vi "CG-Test.vi"() -> ()   [LabVIEW 2020, in "Erweiterte Konfig.lvlib" / "CG-Check Konfig.lvlib"]
uses:
  CG-Check Konfig.lvlib
  Visualisierungs Elemente/String - Ausgabefeld.ctl
  Aktion_CG-Check.ctl
  Aktion_CG-Check_Protokoll.ctl
  CalEingaenge.ctl
  Zustand CG-Check.ctl
  Funktionstasten/Funktionstasten-Aktion.ctl
  Funktionstasten/Zustaende.ctl
  CalGas Aufschaltung/FGV CalGas Aktionen.ctl
  Stoerungen/Stoerungen Messgeraet/Aktionen Kommunikation Stoerung.ctl
  FT-IR/FGV FT-IR Gasliste Aktionen.ctl
  Funktionstasten/Freigabe Aktionen.ctl
  Funktionstasten/Funktionstasten.lvlib
  Stoerungen/Stoerungen.lvlib
  Allgemein/allgemeine Sub-VIs.lvlib
  FT-IR/FT-IR.lvlib
  CalGas Aufschaltung/CalGas Aufschaltung.lvlib
panel:
  out "Anzeige 6":string
  out "Istwert 6":sgl format="%#.2f"
  out "Ist\nAbweichung":T1 {"Abweichung 6" format="%#_5g"; "Abweichung 5" format="%#_5g"; "Abweichung 4" format="%#_5g"; "Abweichung 3" format="%#_5g"; "Abweichung 2" format="%#_5g"; "Abweichung 1" format="%#_5g"}
  out "Span Gas":string
  out "Komponenten":T2 {"Komponente 6" items=["---", "NO (350,3000) LP 191C", "NO2 (150) LP 191C (1of2)", "NO2 (2000) LP 191C (2of2)", "N2O (300) LP 191C (1of2)", "NH3 (300) LP 191C (1of2)", "NH3 (900,3000) LP 191C (2of2)", "HNCO (400) 191C", "H2O% (30) LP 191C", "Formaldehyde (70,500) LP 191C", "CO2 low% (4) LP 191C (2of2)", "CO2% (20) LP 191C (1of2)", "CO (700) LP 191C (1of3)", "CO% (1) LP 191C (2of3)", "Propylene (1000) LP 191C", "Aromatic HC C7 (500) LP 191C", "Ethylene (1000) LP 191C", "CH4 (250) LP 191C (1of2)", "CH4 (5000) LP 191C (2of2)", "Ethane (1000) LP 191C", "Acetylene (1000) LP 191C", "HNO2 (20) 191C", "MeOH (1000) 191C", "CO% (10) LP 191C (3of3)", "Formic Acid (100) 191C", "SO2 (500) LP 191C", "Acetaldehyde (1000) LP 191C", "COS (100) LP 191C", "1,3 butadiene (100) LP 191C", "Oil as Octane (200) LP 191C", "N2O (1000) LP 191C (2of2)", "Propane (200) LP 191C", "NO2 autorange (2000)", "CO autorange (100000)", "CH4 autorange (5000)", "NH3 autorange (3000)", "NOx autorange (3000)", "HCD (10000)", "NMHCD (10000)", "CO2% autorange (20)", "H2Oppm (300000)", "N2O autorange (1000)", "NMNEHCD (3000)", "FEQTHC ppmC1", "Temp. Gascell", "Pressure Gascell", "sBeam@2500", "Temp. HL to FT-IR", "Temp. HL Extern SP1", "Outlet Temp FT-IR", "Temp. Cabinet", "Constant 0", "Constant 50", "Constant 100", "AK DUMMY"]; "Komponente 5" items=["---", "NO (350,3000) LP 191C", "NO2 (150) LP 191C (1of2)", "NO2 (2000) LP 191C (2of2)", "N2O (300) LP 191C (1of2)", "NH3 (300) LP 191C (1of2)", "NH3 (900,3000) LP 191C (2of2)", "HNCO (400) 191C", "H2O% (30) LP 191C", "Formaldehyde (70,500) LP 191C", "CO2 low% (4) LP 191C (2of2)", "CO2% (20) LP 191C (1of2)", "CO (700) LP 191C (1of3)", "CO% (1) LP 191C (2of3)", "Propylene (1000) LP 191C", "Aromatic HC C7 (500) LP 191C", "Ethylene (1000) LP 191C", "CH4 (250) LP 191C (1of2)", "CH4 (5000) LP 191C (2of2)", "Ethane (1000) LP 191C", "Acetylene (1000) LP 191C", "HNO2 (20) 191C", "MeOH (1000) 191C", "CO% (10) LP 191C (3of3)", "Formic Acid (100) 191C", "SO2 (500) LP 191C", "Acetaldehyde (1000) LP 191C", "COS (100) LP 191C", "1,3 butadiene (100) LP 191C", "Oil as Octane (200) LP 191C", "N2O (1000) LP 191C (2of2)", "Propane (200) LP 191C", "NO2 autorange (2000)", "CO autorange (100000)", "CH4 autorange (5000)", "NH3 autorange (3000)", "NOx autorange (3000)", "HCD (10000)", "NMHCD (10000)", "CO2% autorange (20)", "H2Oppm (300000)", "N2O autorange (1000)", "NMNEHCD (3000)", "FEQTHC ppmC1", "Temp. Gascell", "Pressure Gascell", "sBeam@2500", "Temp. HL to FT-IR", "Temp. HL Extern SP1", "Outlet Temp FT-IR", "Temp. Cabinet", "Constant 0", "Constant 50", "Constant 100", "AK DUMMY"]; "Komponente 4" items=["---", "NO (350,3000) LP 191C", "NO2 (150) LP 191C (1of2)", "NO2 (2000) LP 191C (2of2)", "N2O (300) LP 191C (1of2)", "NH3 (300) LP 191C (1of2)", "NH3 (900,3000) LP 191C (2of2)", "HNCO (400) 191C", "H2O% (30) LP 191C", "Formaldehyde (70,500) LP 191C", "CO2 low% (4) LP 191C (2of2)", "CO2% (20) LP 191C (1of2)", "CO (700) LP 191C (1of3)", "CO% (1) LP 191C (2of3)", "Propylene (1000) LP 191C", "Aromatic HC C7 (500) LP 191C", "Ethylene (1000) LP 191C", "CH4 (250) LP 191C (1of2)", "CH4 (5000) LP 191C (2of2)", "Ethane (1000) LP 191C", "Acetylene (1000) LP 191C", "HNO2 (20) 191C", "MeOH (1000) 191C", "CO% (10) LP 191C (3of3)", "Formic Acid (100) 191C", "SO2 (500) LP 191C", "Acetaldehyde (1000) LP 191C", "COS (100) LP 191C", "1,3 butadiene (100) LP 191C", "Oil as Octane (200) LP 191C", "N2O (1000) LP 191C (2of2)", "Propane (200) LP 191C", "NO2 autorange (2000)", "CO autorange (100000)", "CH4 autorange (5000)", "NH3 autorange (3000)", "NOx autorange (3000)", "HCD (10000)", "NMHCD (10000)", "CO2% autorange (20)", "H2Oppm (300000)", "N2O autorange (1000)", "NMNEHCD (3000)", "FEQTHC ppmC1", "Temp. Gascell", "Pressure Gascell", "sBeam@2500", "Temp. HL to FT-IR", "Temp. HL Extern SP1", "Outlet Temp FT-IR", "Temp. Cabinet", "Constant 0", "Constant 50", "Constant 100", "AK DUMMY"]; "Komponente 3" items=["---", "NO (350,3000) LP 191C", "NO2 (150) LP 191C (1of2)", "NO2 (2000) LP 191C (2of2)", "N2O (300) LP 191C (1of2)", "NH3 (300) LP 191C (1of2)", "NH3 (900,3000) LP 191C (2of2)", "HNCO (400) 191C", "H2O% (30) LP 191C", "Formaldehyde (70,500) LP 191C", "CO2 low% (4) LP 191C (2of2)", "CO2% (20) LP 191C (1of2)", "CO (700) LP 191C (1of3)", "CO% (1) LP 191C (2of3)", "Propylene (1000) LP 191C", "Aromatic HC C7 (500) LP 191C", "Ethylene (1000) LP 191C", "CH4 (250) LP 191C (1of2)", "CH4 (5000) LP 191C (2of2)", "Ethane (1000) LP 191C", "Acetylene (1000) LP 191C", "HNO2 (20) 191C", "MeOH (1000) 191C", "CO% (10) LP 191C (3of3)", "Formic Acid (100) 191C", "SO2 (500) LP 191C", "Acetaldehyde (1000) LP 191C", "COS (100) LP 191C", "1,3 butadiene (100) LP 191C", "Oil as Octane (200) LP 191C", "N2O (1000) LP 191C (2of2)", "Propane (200) LP 191C", "NO2 autorange (2000)", "CO autorange (100000)", "CH4 autorange (5000)", "NH3 autorange (3000)", "NOx autorange (3000)", "HCD (10000)", "NMHCD (10000)", "CO2% autorange (20)", "H2Oppm (300000)", "N2O autorange (1000)", "NMNEHCD (3000)", "FEQTHC ppmC1", "Temp. Gascell", "Pressure Gascell", "sBeam@2500", "Temp. HL to FT-IR", "Temp. HL Extern SP1", "Outlet Temp FT-IR", "Temp. Cabinet", "Constant 0", "Constant 50", "Constant 100", "AK DUMMY"]; "Komponente 2" items=["---", "NO (350,3000) LP 191C", "NO2 (150) LP 191C (1of2)", "NO2 (2000) LP 191C (2of2)", "N2O (300) LP 191C (1of2)", "NH3 (300) LP 191C (1of2)", "NH3 (900,3000) LP 191C (2of2)", "HNCO (400) 191C", "H2O% (30) LP 191C", "Formaldehyde (70,500) LP 191C", "CO2 low% (4) LP 191C (2of2)", "CO2% (20) LP 191C (1of2)", "CO (700) LP 191C (1of3)", "CO% (1) LP 191C (2of3)", "Propylene (1000) LP 191C", "Aromatic HC C7 (500) LP 191C", "Ethylene (1000) LP 191C", "CH4 (250) LP 191C (1of2)", "CH4 (5000) LP 191C (2of2)", "Ethane (1000) LP 191C", "Acetylene (1000) LP 191C", "HNO2 (20) 191C", "MeOH (1000) 191C", "CO% (10) LP 191C (3of3)", "Formic Acid (100) 191C", "SO2 (500) LP 191C", "Acetaldehyde (1000) LP 191C", "COS (100) LP 191C", "1,3 butadiene (100) LP 191C", "Oil as Octane (200) LP 191C", "N2O (1000) LP 191C (2of2)", "Propane (200) LP 191C", "NO2 autorange (2000)", "CO autorange (100000)", "CH4 autorange (5000)", "NH3 autorange (3000)", "NOx autorange (3000)", "HCD (10000)", "NMHCD (10000)", "CO2% autorange (20)", "H2Oppm (300000)", "N2O autorange (1000)", "NMNEHCD (3000)", "FEQTHC ppmC1", "Temp. Gascell", "Pressure Gascell", "sBeam@2500", "Temp. HL to FT-IR", "Temp. HL Extern SP1", "Outlet Temp FT-IR", "Temp. Cabinet", "Constant 0", "Constant 50", "Constant 100", "AK DUMMY"]; "Komponente 1" items=["---", "NO (350,3000) LP 191C", "NO2 (150) LP 191C (1of2)", "NO2 (2000) LP 191C (2of2)", "N2O (300) LP 191C (1of2)", "NH3 (300) LP 191C (1of2)", "NH3 (900,3000) LP 191C (2of2)", "HNCO (400) 191C", "H2O% (30) LP 191C", "Formaldehyde (70,500) LP 191C", "CO2 low% (4) LP 191C (2of2)", "CO2% (20) LP 191C (1of2)", "CO (700) LP 191C (1of3)", "CO% (1) LP 191C (2of3)", "Propylene (1000) LP 191C", "Aromatic HC C7 (500) LP 191C", "Ethylene (1000) LP 191C", "CH4 (250) LP 191C (1of2)", "CH4 (5000) LP 191C (2of2)", "Ethane (1000) LP 191C", "Acetylene (1000) LP 191C", "HNO2 (20) 191C", "MeOH (1000) 191C", "CO% (10) LP 191C (3of3)", "Formic Acid (100) 191C", "SO2 (500) LP 191C", "Acetaldehyde (1000) LP 191C", "COS (100) LP 191C", "1,3 butadiene (100) LP 191C", "Oil as Octane (200) LP 191C", "N2O (1000) LP 191C (2of2)", "Propane (200) LP 191C", "NO2 autorange (2000)", "CO autorange (100000)", "CH4 autorange (5000)", "NH3 autorange (3000)", "NOx autorange (3000)", "HCD (10000)", "NMHCD (10000)", "CO2% autorange (20)", "H2Oppm (300000)", "N2O autorange (1000)", "NMNEHCD (3000)", "FEQTHC ppmC1", "Temp. Gascell", "Pressure Gascell", "sBeam@2500", "Temp. HL to FT-IR", "Temp. HL Extern SP1", "Outlet Temp FT-IR", "Temp. Cabinet", "Constant 0", "Constant 50", "Constant 100", "AK DUMMY"]}
  out "Anzeige 5":string
  out "Anzeige 4":string
  out "Anzeige 3":string
  out "Anzeige 2":string
  out "Anzeige 1":string
  out "max.\nAbweichung":T1 {"Abweichung 6" format="%#_5g"; "Abweichung 5" format="%#_5g"; "Abweichung 4" format="%#_5g"; "Abweichung 3" format="%#_5g"; "Abweichung 2" format="%#_5g"; "Abweichung 1" format="%#_5g"}
  out "Sollwerte":T3 caption="Sollwert" {"Sollwert 6" format="%#.3f"; "Sollwert 5" format="%#.3f"; "Sollwert 4" format="%#.3f"; "Sollwert 3" format="%#.3f"; "Sollwert 2" format="%#.3f"; "Sollwert 1" format="%#.3f"}
  out "Zeitanzeige":string
  out "Counter":sgl caption="sec"
  in  "Beenden":bool
  out "Ausgabefeld":T4
  out "Istwert 5":sgl format="%#.2f"
  out "Istwert 4":sgl format="%#.2f"
  out "Istwert 3":sgl format="%#.2f"
  out "Istwert 2":sgl format="%#.2f"
  out "Istwert 1":sgl caption="ppm" format="%#.2f"
  # "Cal Gas - Test"
  # "Istwert"
  # "Komponente"
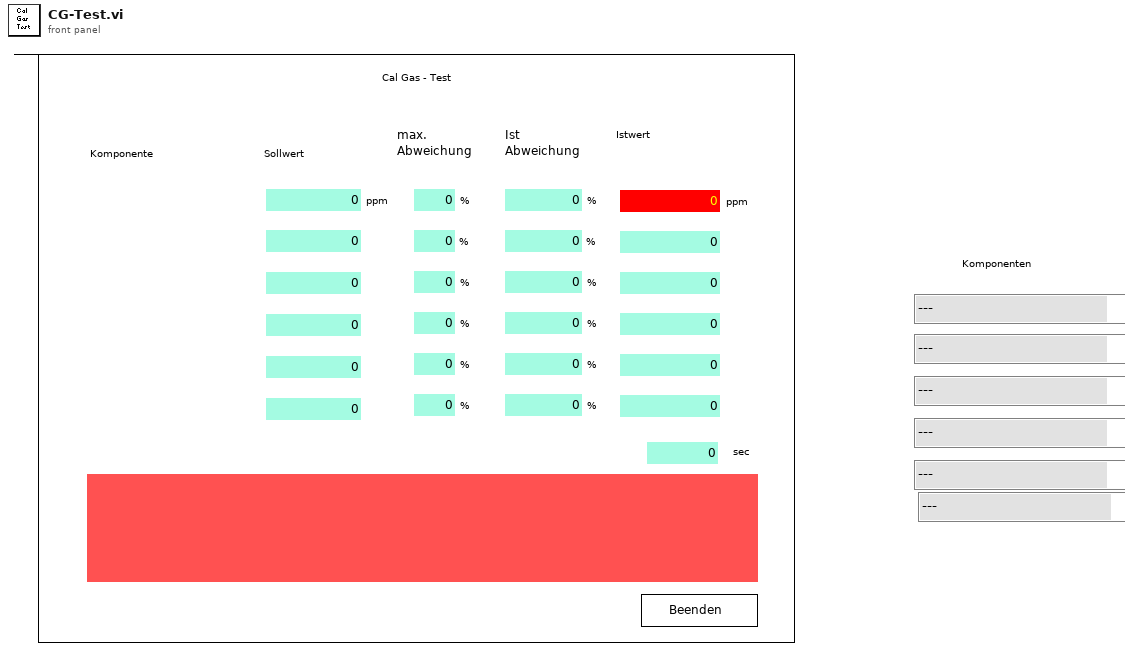
[diagram p1: front panel]
types:
  T1 = cluster{"Abweichung 1":sgl, "Abweichung 2":sgl, "Abweichung 3":sgl, "Abweichung 4":sgl, "Abweichung 5":sgl, "Abweichung 6":sgl}
  T2 = cluster{"Komponente 1":u16, "Komponente 2":u16, "Komponente 3":u16, "Komponente 4":u16, "Komponente 5":u16, "Komponente 6":u16}
  T3 = cluster{"Sollwert 1":sgl, "Sollwert 2":sgl, "Sollwert 3":sgl, "Sollwert 4":sgl, "Sollwert 5":sgl, "Sollwert 6":sgl}
  T4 = typedef "String - Ausgabefeld.ctl" = string
  T5 = typedef "Erweiterte Konfig.lvlib/CG-Check Konfig.lvlib/Aktion_CG-Check.ctl" = enum16{"lesen", "schreiben", "laden", "Komponente", "Aktive?", "speichern"}
  T6 = typedef "Auswahlfeld.ctl" = u16
  T7 = typedef "Erweiterte Konfig.lvlib/CG-Check Konfig.lvlib/Aktion_CG-Check_Protokoll.ctl" = enum16{"Zeitstempel", "Sollwerte", "Istwerte", "Vorzeitig beendet", "Auswerten", "Speichern", "Lesen"}
  T8 = typedef "Erweiterte Konfig.lvlib/CG-Check Konfig.lvlib/CalEingaenge.ctl" = string[]
  T9 = typedef "Funktionstasten.lvlib/Funktionstasten-Aktion.ctl" = enum16{"Initialisieren", "Zustand setzen", "Taste gedrückt", "Fehler speichern", "Lesen", "Manuell", "Remote", "Bitparallel", "Samplepoint", "Zeit Prüfen", "reset Umschalten"}
  T10 = typedef "CalGas Aufschaltung.lvlib/FGV CalGas Aktionen.ctl" = enum16{"lesen", "Analysator Auswahl", "Def.CalGas", "Aufschaltung CalGas", "laden", "speichern", "KAL extrahieren"}
  T11 = typedef "Funktionstasten.lvlib/Zustaende.ctl" = enum16{"Standby", "Pause", "Eco", "Messen", "Kalibrieren", "Spülen Filter", "Spülen Leitung", "Umgebungsluft", "0-Gas", "Cal-Gas", "CG zu PNS", "-------------", "Init 1", "Init 2", "Init 3", "Init 4", "Messen vorbereiten", "Messen durchführen", "Exit"}
  T12 = typedef "Stoerungen.lvlib/Aktionen Kommunikation Stoerung.ctl" = enum16{"lesen", "init", "FT-IR Komm", "FT-IR Betriebsart", "FT-IR Hintergrund", "cRIO Komm", "PNS Komm", "Dichtheitstest", "Life Bit", "FTIR Komm AK", "PMA Komm", "FID Komm", "PMA Cal", "FID Ch4 Cal", "FID THC Cal", "Cal Timeout", "VFS 1 Komm", "VFS 2 Komm", "VFS 3 Komm", "VFS 4 Komm", "TRE 08 Komm", "CG-Test vorzeitig", "CG-Test Span 1", "CG-Test Span 2", "CG-Test Span 3", "CG-Test Messgas", "CG-Test löschen", "Test", "Amium AK", "AK Recept konfig", "AK Name konfig", "AK EKFG konfig"}
  T13 = typedef "FT-IR.lvlib/FGV FT-IR Gasliste Aktionen.ctl" = enum16{"lesen", "Gasliste FT-IR", "Gasliste ausgelesen", "laden", "speichern", "löschen"}
  T14 = typedef "Erweiterte Konfig.lvlib/CG-Check Konfig.lvlib/Zustand CG-Check.ctl" = enum16{"Initialisieren", "Aufschaltdauer", "Prüfdauer", "Auswertung", "Fertig"}
  T15 = typedef "CalGas Aufschaltung.lvlib/Aufschaltung CalGas.ctl" = cluster{"Kalibriergas":T6, "Aufschaltpunkt":T16, "Analysator":T17}
  T16 = typedef "CalGas Aufschaltung.lvlib/Auswahl Aufschaltpunkt.ctl" = enum16{"über Filterblock", "Analysator direkt", "über PNS", "Entnahme", "Gasdivider"}
  T17 = typedef "CalGas Aufschaltung.lvlib/Auswahl Analysator.ctl" = enum16{"FT-IR", "FID", "PMA", "PMA/FID/FT-IR"}
  T18 = cluster{"Aufschaltdauer":sgl, "Prüfdauer":sgl, "Mittelwertanzahl":u8}
  T19 = cluster{"Komponenten[0]":u16, "Komponenten[1]":u16, "Komponenten[2]":u16, "Komponenten[3]":u16, "Komponenten[4]":u16, "Komponenten[5]":u16}
  T20 = cluster{"Sollwerte[0]":sgl, "Sollwerte[1]":sgl, "Sollwerte[2]":sgl, "Sollwerte[3]":sgl, "Sollwerte[4]":sgl, "Sollwerte[5]":sgl}
  T21 = cluster{"max Abweichung[0]":sgl, "max Abweichung[1]":sgl, "max Abweichung[2]":sgl, "max Abweichung[3]":sgl, "max Abweichung[4]":sgl, "max Abweichung[5]":sgl}
  T22 = typedef "Funktionstasten.lvlib/Freigabe Aktionen.ctl" = enum16{"prüfen", "Freigabe?", "lesen"}
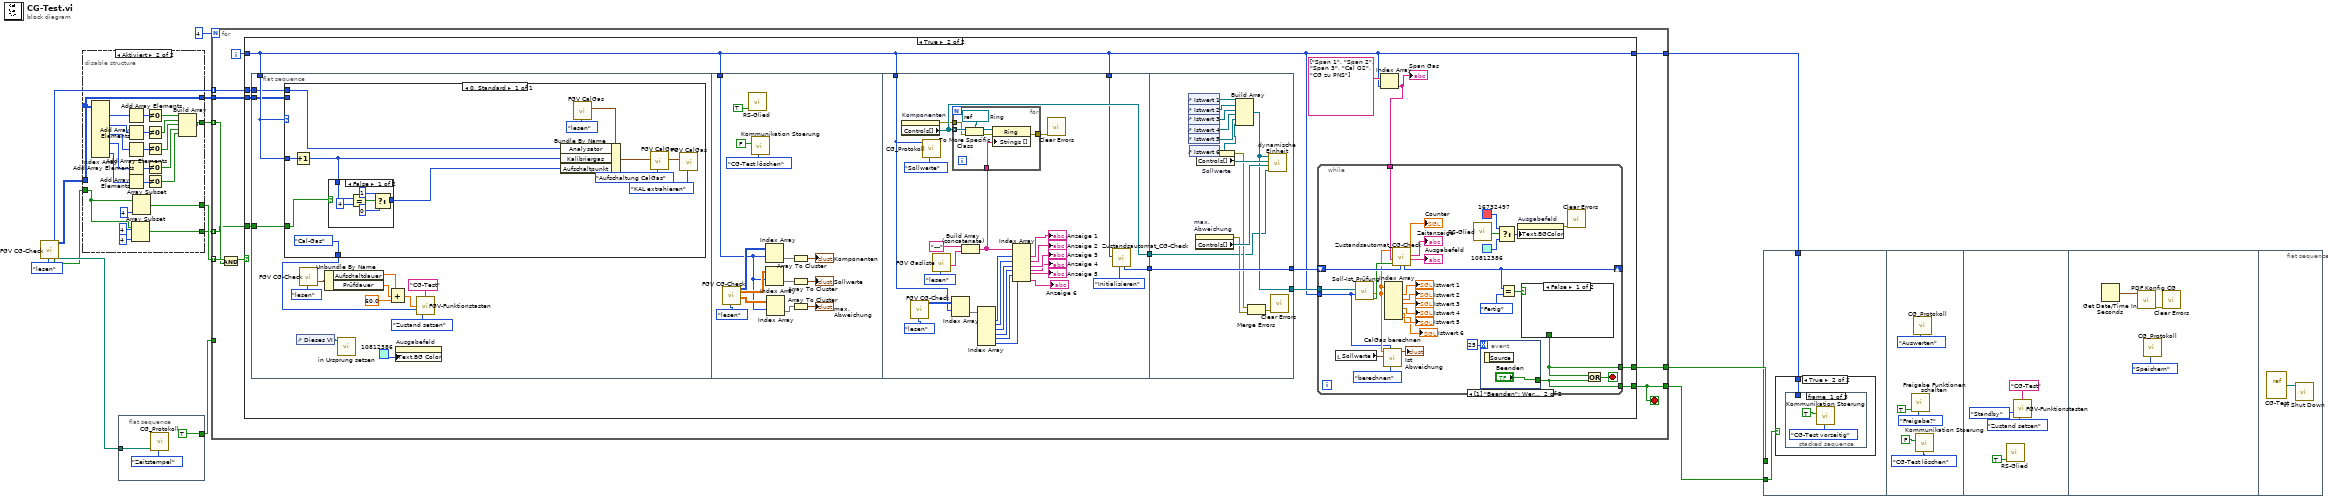
[diagram p0: block diagram]
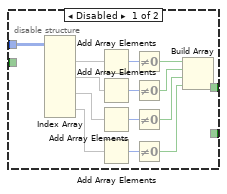
[diagram p2: hidden frame]
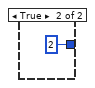
[diagram p4: hidden frame]
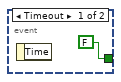
[diagram p5: hidden frame]
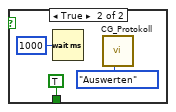
[diagram p6: hidden frame]
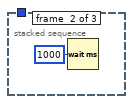
[diagram p8: hidden frame]
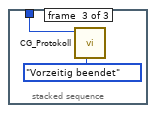
[diagram p9: hidden frame]
diagram:
  n1 = call "FGV CG-Check.vi"("Aktion"=Aktion_CG-Check."lesen") -> ("Analysator"=w1:T6[], "Aktive?"=w5:bool[], "Komponenten"=w12:u16[][], "Pfad:"=w9:path)  [unwired: 11 in, 4 out]
  n2 = disable-structure shown="Aktiviert" {
    disable-tunnel: w12 -> [w28 w38]
    disable-tunnel: [w24 w29] -> w11
    disable-tunnel: w5 -> [_ w30]
    disable-tunnel: [_ w39] -> w3
    disable-tunnel: [_ w38] -> w4
    disable-tunnel: [_ w31] -> w2
    frame Disabled {
      n3 = Index Array(array=w28) -> (element #1=w27:u16[], element #2=w21:u16[], element #3=w20:u16[], element #4=w15:u16[])  [unwired: 8 in]
      n4 = Add Array Elements(numeric array=w27) -> (sum=w26:u16)
      n5 = Add Array Elements(numeric array=w21) -> (sum=w23:u16)
      n6 = Add Array Elements(numeric array=w20) -> (sum=w22:u16)
      n7 = Add Array Elements(numeric array=w15) -> (sum=w17:u16)
      n8 = Not Equal To 0?(x=w26) -> (x != 0?=w25:bool)
      n9 = Not Equal To 0?(x=w23) -> (x != 0?=w19:bool)
      n10 = Not Equal To 0?(x=w22) -> (x != 0?=w18:bool)
      n11 = Not Equal To 0?(x=w17) -> (x != 0?=w16:bool)
      n12 = Build Array(w25, w19, w18, w16) -> (w24:bool[])
    }
    frame Enabled {
      n13 = Index Array(array=w38) -> (element #1=w51:u16[], element #2=w46:u16[], element #3=w45:u16[], element #4=w40:u16[], element #5=w36:u16[])  [unwired: 10 in]
      n14 = Add Array Elements(numeric array=w51) -> (sum=w50:u16)
      n15 = Add Array Elements(numeric array=w46) -> (sum=w48:u16)
      n16 = Add Array Elements(numeric array=w45) -> (sum=w47:u16)
      n17 = Add Array Elements(numeric array=w40) -> (sum=w42:u16)
      n18 = Add Array Elements(numeric array=w36) -> (sum=w37:u16)
      n19 = Array Subset(array=w30, index=4 ("Index"), length=4 ("Länge")) -> (w31:bool[])
      n20 = Array Subset(array=w30, length=4 ("Länge")) -> (w29:bool[])  [unwired: 1 in]
      n21 = Not Equal To 0?(x=w50) -> (x != 0?=w49:bool)
      n22 = Not Equal To 0?(x=w48) -> (x != 0?=w44:bool)
      n23 = Not Equal To 0?(x=w47) -> (x != 0?=w43:bool)
      n24 = Not Equal To 0?(x=w42) -> (x != 0?=w41:bool)
      n25 = Not Equal To 0?(x=w37) -> (x != 0?=w35:bool)
      n26 = Build Array(w49, w44, w43, w41, w35) -> (w39:bool[])
    }
  }
  n27 = flat-sequence {
    tunnel: [TRUE] -> w10
    tunnel: w9 -> [w52]
    frame #0 {
      n28 = call "CG_Protokoll.vi"("Aktion"=Aktion_CG-Check_Protokoll."Zeitstempel", "Pfad"=w52) -> ()  [unwired: 8 in, 2 out]
    }
  }
  n29 = for {
    N: 4 -> [_]
    tunnel: [w64] -> w14
    tunnel: w11 -> [w59] mode=indexing
    tunnel: w10 -> [_]
    tunnel: [w62] -> w7
    tunnel: [w61] -> w6
    tunnel: w4 -> [w60]
    tunnel: w3 -> [w57] mode=indexing
    tunnel: w2 -> [w56] mode=indexing
    tunnel: w1 -> [w55] mode=indexing
    i -> [w63]
    stop <- w62 stop-if-true
    n30 = And(x=w59, y=w57) -> (x .and. y?=w58:bool)
    n31 = case shown="True" w58 {
      tunnel: [_ w74] -> w64
      tunnel: w63 -> [_ w69]
      tunnel: [_ w71] -> w62
      tunnel: [_ w69] -> w61
      tunnel: w60 -> [_ w67]
      tunnel: w56 -> [_ w66]
      tunnel: w55 -> [_ w65]
      frame False {
      }
      frame True {
        n32 = flat-sequence {
          tunnel: w69 -> [w81]
          tunnel: w67 -> [w79]
          tunnel: w66 -> [w78]
          tunnel: w65 -> [w77]
          tunnel: w69 -> [w111]
          tunnel: [w150] -> w76
          tunnel: [w141] -> w75
          tunnel: w69 -> [w130]
          tunnel: w69 -> [w127]
          tunnel: [w172] -> w73
          tunnel: w76 -> [w172]
          tunnel: w75 -> [w159]
          tunnel: [w164] -> w72
          frame #0 {
            n33 = case shown="0, Standard" w81 {
              tunnel: w81 -> [w103]
              tunnel: [Zustaende."Cal-Gas" ("Zustand")] -> w80
              tunnel: w79 -> [_]
              tunnel: w78 -> [w93]
              tunnel: w77 -> [w92]
              frame 0, Default {
                n34 = Increment(x=w103) -> (x+1=w95:i32)
                n35 = case shown="False" w93 {
                  tunnel: w95 -> [w109 _]
                  tunnel: [w104 2 ("f")] -> w94
                  frame False {
                    n36 = Equal?(x=w109, y=4) -> (x = y?=w107:bool)
                    n37 = Select(t=1, s=w107, f=0) -> (s? t:f=w104:i32)
                  }
                  frame True {
                  }
                }
                n38 = call "FGV CalGas.vi"("Aktionen"=FGV_CalGas_Aktionen."lesen") -> ("Aufschaltung CalGas"=w99:T15)  [unwired: 6 in, 4 out]
                n39 = Bundle By Name(cluster=w99, "Analysator"=w92, "Kalibriergas"=w95, "Aufschaltpunkt"=w94) -> (w101:T15)
                n40 = call "FGV CalGas.vi"("Aktionen"=FGV_CalGas_Aktionen."Aufschaltung CalGas", "Aufschaltung CalGas"=w101) -> ("Aufschaltung CalGas"=w97:T15)  [unwired: 5 in, 4 out]
                n41 = call "FGV CalGas.vi"("Aktionen"=FGV_CalGas_Aktionen."KAL extrahieren", "Aufschaltung CalGas"=w97) -> ()  [unwired: 5 in, 5 out]
              }
            }
            n42 = control-ref of="Dieses VI"() -> (w82:refnum<vi>)
            n43 = call "FGV CG-Check.vi"("Aktion"=Aktion_CG-Check."lesen") -> ("Cluster"=w89:T18)  [unwired: 11 in, 7 out]
            n44 = Unbundle By Name(w89) -> ("Aufschaltdauer"=w85:sgl, "Prüfdauer"=w84:sgl)
            n45 = call "in Ursprung setzen.vi"("VI Referenz"=w82) -> ()  [unwired: 10 in, 1 out]
            n46 = Compound Arithmetic op=ADD(w85, w84, sgl 60.0 ("Wert")) -> (w91:sgl)
            n47 = property on="Ausgabefeld" class="Str (strikt)"("Text.BG Color"=u32 10812386) -> ()  [unwired: 2 in, 2 out]
            n48 = call "FGV-Funktionstasten.vi"("Herkunft"="CG-Test", "Zeit"=w91, "Zustand"=w80, "Aktion"=Funktionstasten-Aktion."Zustand setzen") -> ()  [unwired: 4 in, 8 out]
          }
          frame #1 {
            n49 = call "FGV CG-Check.vi"("Aktion"=Aktion_CG-Check."lesen") -> ("Komponenten"=w116:u16[][], "Sollwerte"=w115:sgl[][], "max Abweichung"=w113:sgl[][])  [unwired: 11 in, 5 out]
            n50 = call "RS-Glied.vi"("reset"=TRUE) -> ()  [unwired: 10 in, 1 out]
            n51 = call "Kommunikation Stoerung.vi"("Aktionen"=Aktionen_Kommunikation_Stoerung."CG-Test löschen", "ERROR"=FALSE) -> ()  [unwired: 9 in, 1 out]
            n52 = Index Array(array=w116, index (row)=w111) -> (element=w117:u16[])  [unwired: 1 in]
            n53 = Index Array(array=w115, index (row)=w111) -> (element=w114:sgl[])  [unwired: 1 in]
            n54 = Index Array(array=w113, index (row)=w111) -> (element=w112:sgl[])  [unwired: 1 in]
            n55 = Array To Cluster(array=w117) -> (cluster=→"Komponenten":T19)
            n56 = Array To Cluster(array=w114) -> (cluster=→"Sollwerte":T20)
            n57 = Array To Cluster(array=w112) -> (cluster=→"max.\nAbweichung":T21)
          }
          frame #2 {
            n58 = property on="Komponenten" class="Cluster (strikt)"() -> (error out=w139:errorcluster, "Controls[]"=w141:refnum<vi>[])  [unwired: 2 in, 1 out]
            n59 = call "FGV CG-Check.vi"("Aktion"=Aktion_CG-Check."lesen") -> ("Komponenten"=w138:u16[][])  [unwired: 11 in, 7 out]
            n60 = call "CG_Protokoll.vi"("Aktion"=Aktion_CG-Check_Protokoll."Sollwerte", "Index"=w130) -> ()  [unwired: 8 in, 2 out]
            n61 = call "FGV Gasliste.vi"("Aktionen"=FGV_FT-IR_Gasliste_Aktionen."lesen") -> ("Aktuelle Gasliste gesamt"=w137:T4[])  [unwired: 8 in, 2 out]
            n62 = Index Array(array=w138, index (row)=w130) -> (element=w136:u16[])  [unwired: 1 in]
            n63 = Build Array (concatenate)("---", w137) -> (w143:T4[])
            n64 = for {
              tunnel: w141 -> [w158] mode=indexing
              tunnel: w143 -> [w152]
              tunnel: [w154] -> w140
              tunnel: w139 -> [w153]
              w157 = refnum<vi> refnum  # Ring
              n65 = To More Specific Class(target class=w157, reference=w158, error in=w153) -> (specific class reference=w156:refnum<vi>, error out=w155:errorcluster)
              n66 = property class="Ring"(reference=w156, error in=w155, "Strings []"=w152) -> (error out=w154:errorcluster)  [unwired: 1 out]
            }
            n67 = Index Array(array=w136) -> (element #1=w135:u16, element #2=w134:u16, element #3=w133:u16, element #4=w132:u16, element #5=w131:u16, element #6=w125:u16)  [unwired: 6 in]
            n68 = Index Array(array=w143, index #1=w135, index #2=w134, index #3=w133, index #4=w132, index #5=w131, index #6=w125) -> (element #1=→"Anzeige 1":T4, element #2=→"Anzeige 2":T4, element #3=→"Anzeige 3":T4, element #4=→"Anzeige 4":T4, element #5=→"Anzeige 5":T4, element #6=→"Anzeige 6":T4)
            n69 = call <vilib>:"Clear Errors.vi"("error in (no error)"=w140) -> ()  [unwired: 5 in, 2 out]
            n70 = call "Zustandsautomat_CG-Check.vi"("Zustand"=Zustand_CG-Check."Initialisieren", "Index"=w127) -> ("Zustand"=w150:T14)  [unwired: 5 in, 4 out]
          }
          frame #3 {
            n71 = control-ref of="Istwert 1"() -> (w171:refnum<vi>)
            n72 = control-ref of="Istwert 2"() -> (w170:refnum<vi>)
            n73 = control-ref of="Istwert 3"() -> (w169:refnum<vi>)
            n74 = control-ref of="Istwert 4"() -> (w168:refnum<vi>)
            n75 = control-ref of="Istwert 5"() -> (w167:refnum<vi>)
            n76 = control-ref of="Istwert 6"() -> (w160:refnum<vi>)
            n77 = property on="max.\nAbweichung" class="Cluster (strikt)"() -> (error out=w162:errorcluster, "Controls[]"=w166:refnum<vi>[])  [unwired: 2 in, 1 out]
            n78 = property on="Sollwerte" class="Cluster (strikt)"() -> (error out=w163:errorcluster, "Controls[]"=w165:refnum<vi>[])  [unwired: 2 in, 1 out]
            n79 = Build Array(w171, w170, w169, w168, w167, w160) -> (w164:refnum<vi>[])
            n80 = Merge Errors(w163, w162) -> (w161:errorcluster)
            n81 = call "dynamische Einheit.vi"("Komponenten Ref."=w159, "max.Abweichung Ref."=w166, "Sollwert Ref."=w165, "Istwerte Ref."=w164) -> ()  [unwired: 8 in]
            n82 = call <vilib>:"Clear Errors.vi"("error in (no error)"=w161) -> ()  [unwired: 5 in, 2 out]
          }
        }
        n83 = Index Array(array=T8 ["Span 1", "Span 2", "Span 3", "Cal O2", "CG zu PNS"], index=w69) -> (element=w68:string)
        "Span Gas" <- w68
        n84 = while {
          shift-right: [w201] -> _
          shift-left: w73 -> [w202]
          tunnel: [w183] -> w74
          tunnel: w72 -> [w174]
          tunnel: w69 -> [w175]
          tunnel: w68 -> [w200]
          tunnel: [w180] -> w71
          stop <- w182 stop-if-true
          n85 = local read "Sollwerte"() -> (w178:T3)
          n86 = call "Soll-Ist_Prüfung.vi"("Index"=w175, "Istwerte Ref."=w174) -> ("Fehler"=w185:bool, "Istwert"=w179:sgl[])  [unwired: 8 in]
          n87 = call "CalGas berechnen.vi"("Aktion"=enum16{"lesen", "berechnen"}."berechnen", "Index"=w175, "Sollwerte"=w178, "Istwert"=w179) -> ("Ist\nAbweichung"=→"Ist\nAbweichung":T1)  [unwired: 5 in, 2 out]
          n88 = Index Array(array=w179) -> (element #1=→"Istwert 1":sgl, element #2=→"Istwert 2":sgl, element #3=→"Istwert 3":sgl, element #4=→"Istwert 4":sgl, element #5=→"Istwert 5":sgl, element #6=→"Istwert 6":sgl)  [unwired: 6 in]
          n89 = call "Zustandsautomat_CG-Check.vi"("Zustand"=w202, "Fehler 2"=w185, "Span Eingang"=w200, "Istwerte"=w179) -> ("Anzeige"=→"Ausgabefeld":string, "Zeitanzeige"=→"Zeitanzeige":string, "Verstrichene Zeit"=→"Counter":sgl, "Zustand"=w201:T14)  [unwired: 3 in, 1 out]
          n90 = call "RS-Glied.vi"() -> ("Fehler"=w186:bool)  [unwired: 11 in]
          n91 = event shown="[1] \"Beenden\": Wertänderung" {
            selector: _ -> [_ _]
            dyn-events: _ -> [_ _]
            timeout: 25 -> [_ _]
            tunnel: [FALSE ("Beenden") "Beenden"] -> w180
            event Timeout {
              n92 = event-data() -> ()  [unwired: 1 in, 1 out]
            }
            event "Beenden": Value Change {
              n93 = event-data() -> ()  [unwired: 1 in, 1 out]
            }
          }
          n94 = Select(t=u32 16732497 ("Hintergrund"), s=w186, f=u32 10812386 ("Hintergrund")) -> (s? t:f=w194:u32)
          n95 = Equal?(x=w201, y=Zustand_CG-Check."Fertig") -> (x = y?=w199:bool)
          n96 = property on="Ausgabefeld" class="Str (strikt)"("Text.BGColor"=w194) -> (error out=w184:errorcluster)  [unwired: 2 in, 1 out]
          n97 = case shown="False" w199 {
            tunnel: [_ TRUE] -> w183
            frame False {
            }
            frame True {
              n98 = Wait (ms)(milliseconds to wait=u32 1000 ("Zu wartende ms")) -> ()  [unwired: 1 out]
              n99 = call "CG_Protokoll.vi"("Aktion"=Aktion_CG-Check_Protokoll."Auswerten") -> ()  [unwired: 9 in, 2 out]
            }
          }
          n100 = call <vilib>:"Clear Errors.vi"("error in (no error)"=w184) -> ()  [unwired: 5 in, 2 out]
          n101 = Or(x=w183, y=w180) -> (x .or. y?=w182:bool)
        }
      }
    }
  }
  n102 = flat-sequence {
    tunnel: w14 -> [_]
    tunnel: w7 -> [w209]
    tunnel: w6 -> [w208]
    frame #0 {
      n103 = case shown="True" w209 {
        tunnel: w208 -> [_ w210]
        frame False {
        }
        frame True {
          n104 = stacked-sequence {
            tunnel: w210 -> [_ _ w214]
            frame #0 {
              n105 = call "Kommunikation Stoerung.vi"("Aktionen"=Aktionen_Kommunikation_Stoerung."CG-Test vorzeitig", "ERROR"=TRUE) -> ()  [unwired: 9 in, 1 out]
            }
            frame #1 {
              n106 = Wait (ms)(milliseconds to wait=u32 1000 ("Zu wartende ms")) -> ()  [unwired: 1 out]
            }
            frame #2 {
              n107 = call "CG_Protokoll.vi"("Aktion"=Aktion_CG-Check_Protokoll."Vorzeitig beendet", "Index"=w214) -> ()  [unwired: 8 in, 2 out]
            }
          }
        }
      }
    }
    frame #1 {
      n108 = call "Freigabe Funktionen schalten.vi"("Aktionen"=Freigabe_Aktionen."Freigabe?", "Freigabe?"=TRUE) -> ()  [unwired: 7 in, 3 out]
      n109 = call "CG_Protokoll.vi"("Aktion"=Aktion_CG-Check_Protokoll."Auswerten") -> ()  [unwired: 9 in, 2 out]
      n110 = call "Kommunikation Stoerung.vi"("Aktionen"=Aktionen_Kommunikation_Stoerung."CG-Test löschen", "ERROR"=FALSE) -> ()  [unwired: 9 in, 1 out]
    }
    frame #2 {
      n111 = call "RS-Glied.vi"("reset"=TRUE) -> ()  [unwired: 10 in, 1 out]
      n112 = call "FGV-Funktionstasten.vi"("Herkunft"="CG-Test", "Zustand"=Zustaende."Standby", "Aktion"=Funktionstasten-Aktion."Zustand setzen") -> ()  [unwired: 5 in, 8 out]
    }
    frame #3 {
      n113 = Get Date/Time In Seconds() -> (seconds since 1Jan1904=w225:timestamp)
      n114 = call "PDF Konfig CG.vi"("seconds since 1Jan1904"=w225) -> ("error out"=w226:errorcluster)  [unwired: 10 in]
      n115 = call "CG_Protokoll.vi"("Aktion"=Aktion_CG-Check_Protokoll."Speichern") -> ()  [unwired: 9 in, 2 out]
      n116 = call <vilib>:"Clear Errors.vi"("error in (no error)"=w226) -> ()  [unwired: 5 in, 2 out]
    }
    frame #4 {
      n117 = vi-ref "CG-Test.vi"() -> (w228:refnum<vi>)
      n118 = call "VI Shut Down.vi"("VI Referenz"=w228) -> ()  [unwired: 11 in]
    }
  }
